vi "Lavi_Ariel_particle_simulation.vi"(9 "Base time interval dt (ms)\n(without compute time)":dbl=30.0 format="%#_13g", 10 "Initial Velocity (boxes/sec)":dbl[](array[numeric]), 11 "Initial Position (boxes)":dbl[](array[numeric])) -> ()   [LabVIEW 2016]
panel:
  in  "Snake length":i32=10
  in  "Force constant (k)":dbl(slide)=10.0 scale=0.1..100.0
  in  "Drag?":bool
  in  "Constant Acceleration?":bool
  out "Acceleration \n(boxes/s^2)":dbl[](array[numeric])
  in  "Coefficient (if true)":dbl(slide)=0.01 scale=0.0001..1.0
  in  "Central Force":T1(ring)=enum."Linear/spring (-kr)" caption="Enum"
  in  "Value (if on/true)":dbl[](array[numeric])=[0.0, -9.8]
  out "Velocity":dbl[](array[numeric])
  out "Position":dbl[](array[numeric])
  in  "stop":bool
  out "dt (ms)":u32
  out "XY Graph":cluster{dbl[], dbl[]}[](graph)
  # "INITIAL CONTROLS"
  # "INDICATORS"
  # "FORCE/ACCELERATION CONTROLS"
  # "Recommended value range:\n1 to 50\n(higher for Coulomb)"
  # "Recommended value range:\n0.001 to 0.01"
  # "Adjust x and y \ncomponents \nmanually"
  # "As stated in the lab manual, I used 2-element arrays to represent position and velocity. I did not make box size adjustable because it is arbitrary. The initial position/velocity must be set manually by entering the x and y components.\n \nThe time interval dt is taken as the output of the Time Since Last Call function (i.e. the base time input + the time it took to complete last iteration of while loop). This ensures that the unit of time is approximately one second.  The extra Time Since Last Call is present just to reset the counter when the code starts. \n\nI recommend a base time input of 15 ms, giving an update rate of 60 fps. Reducing the input more leads to jitteriness, as dt ends up varying by +/- 1 ms. If you want the \"snake\" or \"track\" of points to be more visible, a larger time interval works better."
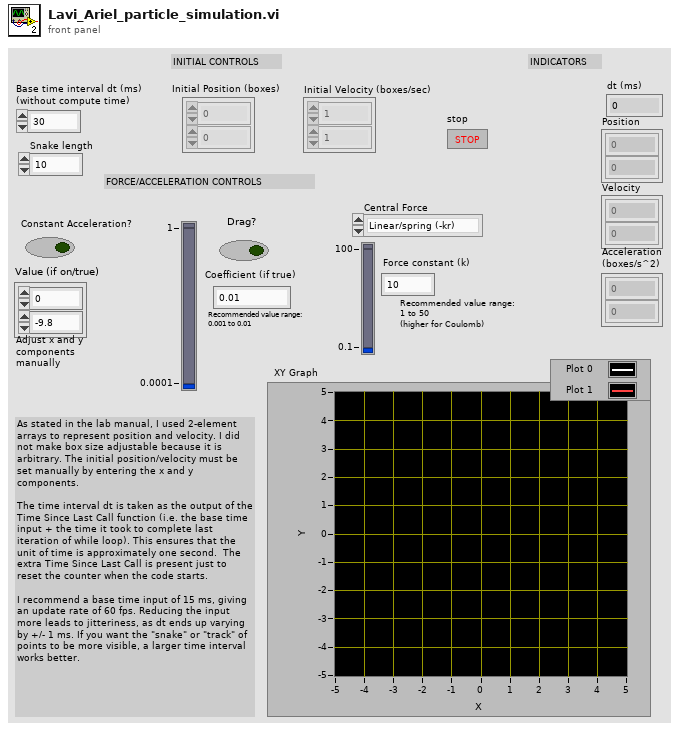
[diagram p1: front panel]
types:
  T1 = enum16{"None", "Coulomb (-k/r^2)", "Linear/spring (-kr)"}
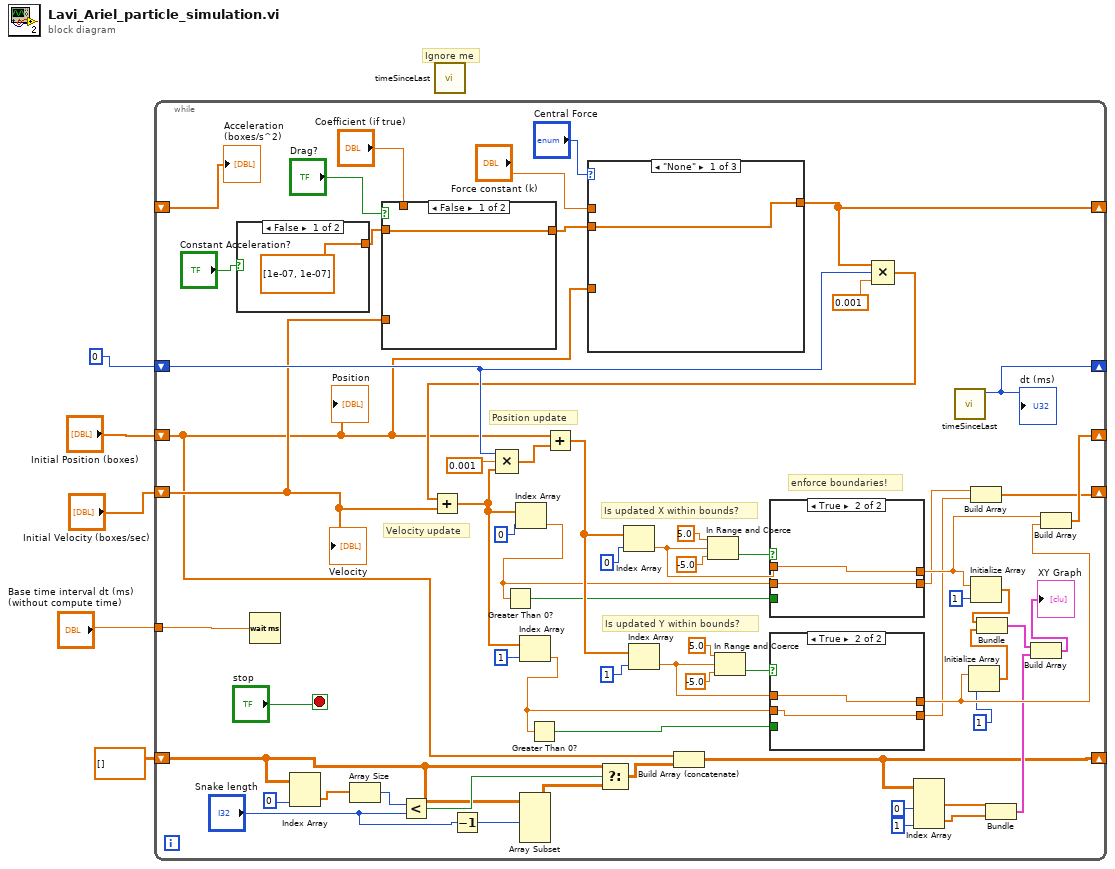
[diagram p0: block diagram]
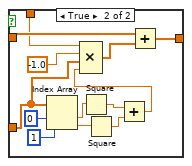
[diagram p2: hidden frame]
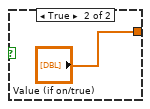
[diagram p3: hidden frame]
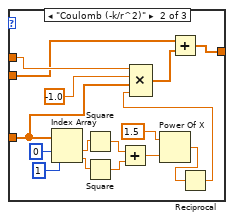
[diagram p4: hidden frame]
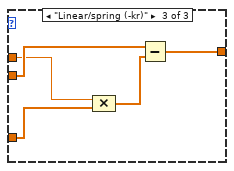
[diagram p5: hidden frame]
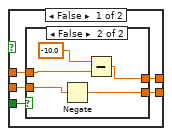
[diagram p6: hidden frame]
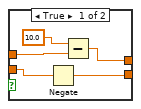
[diagram p7: hidden frame]
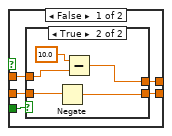
[diagram p8: hidden frame]
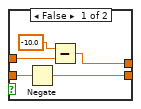
[diagram p9: hidden frame]
diagram:
  # "Ignore me"
  n1 = while {
    shift-right: [w45] -> _
    shift-left: "Initial Position (boxes)" -> [w24]
    shift-right: [w39] -> _
    shift-left: "Initial Velocity (boxes/sec)" -> [w29]
    shift-right: [w68] -> _
    shift-left: u32 0 ("Time since last call") -> [w37]
    tunnel: "Base time interval dt (ms)\n(without compute time)" -> [w67]
    shift-right: [w33] -> _
    shift-left: _ -> [w26]
    shift-right: [w6] -> _
    shift-left: dbl[][] [] -> [w8]
    stop <- "stop" stop-if-true
    # "Velocity update"
    # "Position update"
    # "enforce boundaries!"
    # "Is updated X within bounds?"
    # "Is updated Y within bounds?"
    n2 = case shown="False" "Constant Acceleration?" {
      tunnel: [dbl[] [1e-07, 1e-07] ("Value (if on/true) 2") "Value (if on/true)"] -> w31
      frame False {
      }
      frame True {
      }
    }
    n3 = Wait (ms)(milliseconds to wait=w67) -> ()  [unwired: 1 out]
    n4 = Index Array(array=w8, index (col)=0 ("index (row)")) -> (element=w23:dbl[])  [unwired: 1 in]
    n5 = Array Size(array=w23) -> (size(s)=w22:i32)
    n6 = case shown="False" "Drag?" {
      tunnel: w31 -> [w70 w76]
      tunnel: [w70 w77] -> w30
      tunnel: w29 -> [_ w72]
      tunnel: "Coefficient (if true)" -> [_ w71]
      frame False {
      }
      frame True {
        n7 = Index Array(array=w72, index #1=0 ("index"), index #2=1 ("index")) -> (element #1=w74:dbl, element #2=w75:dbl)
        n8 = Square(x=w74) -> (x^2=w81:dbl)
        n9 = Square(x=w75) -> (x^2=w82:dbl)
        n10 = Add(x=w81, y=w82) -> (x+y=w79:dbl)
        n11 = Compound Arithmetic op=MULTIPLY(w71, -1.0 ("value"), w72, w79) -> (w78:dbl[])
        n12 = Add(x=w76, y=w78) -> (x+y=w77:dbl[])
      }
    }
    n13 = Less?(x=w22, y="Snake length") -> (x < y?=w21:bool)
    n14 = Decrement(x="Snake length") -> (x-1=w9:i32)
    n15 = Array Subset(array=w8, length (row)=w9) -> (w20:dbl[][])  [unwired: 3 in]
    n16 = case shown="\"None\"" "Central Force" {
      tunnel: [w86 w93 w106] -> w33
      tunnel: w30 -> [w86 w91 w104]
      tunnel: "Force constant (k)" -> [_ w94 w103]
      tunnel: w24 -> [_ w96 w107]
      frame "None" {
      }
      frame "Coulomb (-k/r^2)" {
        n17 = Index Array(array=w96, index #1=0 ("index"), index #2=1 ("index")) -> (element #1=w97:dbl, element #2=w100:dbl)
        n18 = Square(x=w97) -> (x^2=w99:dbl)
        n19 = Square(x=w100) -> (x^2=w101:dbl)
        n20 = Add(x=w99, y=w101) -> (x+y=w90:dbl)
        n21 = Power Of X(1:w90, 2:1.5) -> (0:w88:dbl)
        n22 = Reciprocal(x=w88) -> (1/x=w87:dbl)
        n23 = Compound Arithmetic op=MULTIPLY(w94, -1.0 ("value"), w96, w87) -> (w92:dbl[])
        n24 = Add(x=w91, y=w92) -> (x+y=w93:dbl[])
      }
      frame "Linear/spring (-kr)" {
        n25 = Compound Arithmetic op=MULTIPLY(w103, w107) -> (w105:dbl[])
        n26 = Subtract(x=w104, y=w105) -> (x-y=w106:dbl[])
      }
    }
    n27 = Select(t=w8, s=w21, f=w20) -> (s? t:f=w7:dbl[][])
    n28 = Build Array (concatenate)(w24, w7) -> (w6:dbl[][])
    n29 = Compound Arithmetic op=MULTIPLY(w33, w37, 0.001 ("value")) -> (w36:dbl[])
    n30 = Add(x=w36, y=w29) -> (x+y=w35:dbl[])
    n31 = Compound Arithmetic op=MULTIPLY(w37, 0.001, w35) -> (w65:dbl[])
    n32 = Index Array(array=w35, index=0) -> (element=w43:dbl)
    n33 = Greater Than 0?(x=w43) -> (x > 0?=w59:bool)
    n34 = Index Array(array=w35, index=1 ("length")) -> (element=w42:dbl)
    n35 = Greater Than 0?(x=w42) -> (x > 0?=w58:bool)
    n36 = Add(x=w24, y=w65) -> (x+y=w63:dbl[])
    n37 = Index Array(array=w63, index=0) -> (element=w51:dbl)
    n38 = Index Array(array=w63, index=1 ("length")) -> (element=w50:dbl)
    n39 = In Range and Coerce(upper limit=5.0, x=w51, lower limit=-5.0 ("upper limit")) -> (In Range?=w57:bool)  [unwired: 1 out]
    n40 = In Range and Coerce(upper limit=5.0, x=w50, lower limit=-5.0) -> (In Range?=w54:bool)  [unwired: 1 out]
    n41 = case shown="True" w57 {
      tunnel: w51 -> [w129 w141]
      tunnel: [w127 w141] -> w47
      tunnel: w59 -> [w128 _]
      tunnel: w43 -> [w126 w140]
      tunnel: [w125 w140] -> w41
      frame False {
        n42 = case shown="True" w128 {
          tunnel: w129 -> [w133 w137]
          tunnel: [w132 w139] -> w127
          tunnel: w126 -> [w131 w136]
          tunnel: [w130 w135] -> w125
          frame False {
            n43 = Negate(x=w131) -> (-x=w130:dbl)
            n44 = Subtract(x=-10.0, y=w133) -> (x-y=w132:dbl)
          }
          frame True {
            n45 = Negate(x=w136) -> (-x=w135:dbl)
            n46 = Subtract(x=10.0, y=w137) -> (x-y=w139:dbl)
          }
        }
      }
      frame True {
      }
    }
    n47 = case shown="True" w54 {
      tunnel: w50 -> [w112 w124]
      tunnel: [w111 w124] -> w46
      tunnel: w58 -> [w110 _]
      tunnel: w42 -> [w109 w123]
      tunnel: [w108 w123] -> w40
      frame False {
        n48 = case shown="False" w110 {
          tunnel: w112 -> [w117 w120]
          tunnel: [w116 w121] -> w111
          tunnel: w109 -> [w114 w119]
          tunnel: [w113 w118] -> w108
          frame True {
            n49 = Negate(x=w114) -> (-x=w113:dbl)
            n50 = Subtract(x=10.0, y=w117) -> (x-y=w116:dbl)
          }
          frame False {
            n51 = Negate(x=w119) -> (-x=w118:dbl)
            n52 = Subtract(x=-10.0, y=w120) -> (x-y=w121:dbl)
          }
        }
      }
      frame True {
      }
    }
    n53 = Index Array(array=w6, index (col) #1=0 ("disabled index (col)"), index (col) #2=1 ("index (col)")) -> (element #1=w15:dbl[], element #2=w14:dbl[])  [unwired: 2 in]
    n54 = call "timeSinceLast.vi"() -> ("Time since last call"=w68:u32)  [unwired: 10 in, 1 out]
    "dt (ms)" <- w68
    n55 = Initialize Array(w46, 1 ("dimension size")) -> (w49:dbl[])
    n56 = Build Array(w41, w40) -> (w39:dbl[])
    n57 = Initialize Array(w47, 1 ("dimension size")) -> (w48:dbl[])
    n58 = Bundle(w48, w49) -> (w11:cluster{dbl[], dbl[]})  [unwired: 1 in]
    n59 = Bundle(w15, w14) -> (w12:cluster{dbl[], dbl[]})  [unwired: 1 in]
    n60 = Build Array(w11, w12) -> (→"XY Graph":cluster{dbl[], dbl[]}[])
    n61 = Build Array(w47, w46) -> (w45:dbl[])
    "Position" <- w24
    "Velocity" <- w29
    "Acceleration \n(boxes/s^2)" <- w26
  }
  n62 = call "timeSinceLast.vi"() -> ()  [unwired: 10 in, 2 out]
